vi "ActorDB-PerformUpdateAllInstruction.vi"(5 "SQL Statement":string, 6 "Cluster Out":T1(array[cluster]), 7 "Update All":bool, 8 "error in (no error)":errorcluster, 9 "Column Number":i32, 10 "Table":string, 11 "Database-API in":refnum<class "Database-API.lvclass">) -> (0 "Error Out":errorcluster[](array[cluster]), 3 "Database-API out":refnum<class "Database-API.lvclass">)   [LabVIEW 2013, in "Database-Actor.lvclass"]
uses:
  Database-Actor.lvclass
  Reuse Library/Database API/Database-API.lvclass
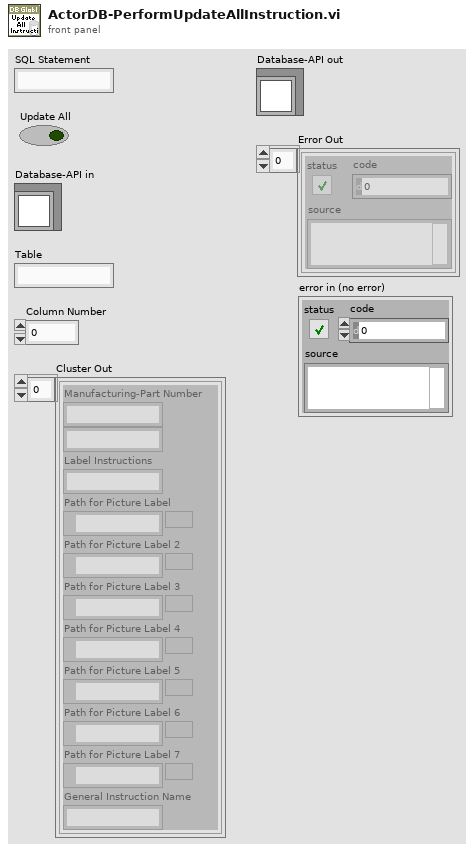
[diagram p1: front panel]
types:
  T1 = cluster{"Manufacturing-Part Number":string, string, "Label Instructions":string, "Path for Picture Label":path, "Path for Picture Label 2":path, "Path for Picture Label 3":path, "Path for Picture Label 4":path, "Path for Picture Label 5":path, "Path for Picture Label 6":path, "Path for Picture Label 7":path, "General Instruction Name":string}[]
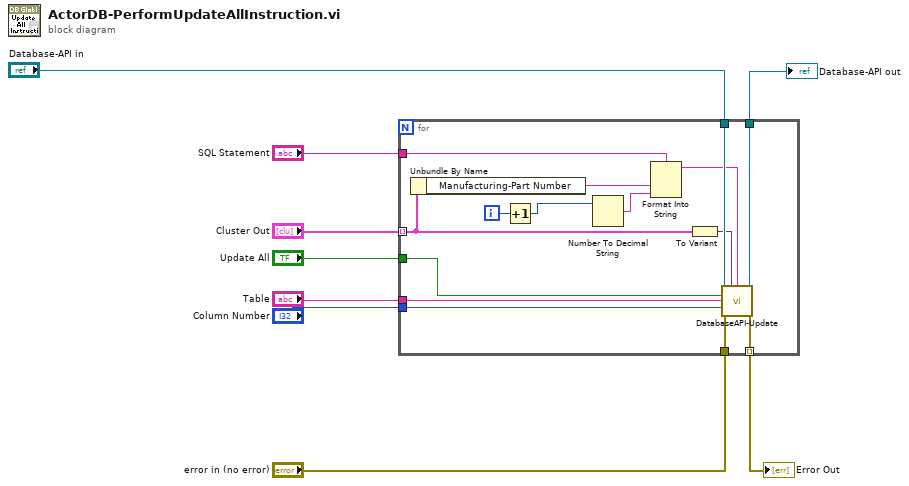
[diagram p0: block diagram]
diagram:
  n1 = for {
    tunnel: "Database-API in" -> [w24]
    tunnel: "Update All" -> [w23]
    tunnel: "SQL Statement" -> [w16]
    tunnel: [w22] -> w4
    tunnel: "Table" -> [w21]
    tunnel: [w20] -> w7 mode=indexing
    tunnel: "Column Number" -> [w19]
    tunnel: "error in (no error)" -> [w18]
    tunnel: "Cluster Out" -> [w15] mode=indexing
    i -> [w13]
    n2 = Unbundle By Name(w15) -> ("Manufacturing-Part Number"=w14:string)
    n3 = Increment(x=w13) -> (x+1=w12:i32)
    n4 = Number To Decimal String(number=w12) -> (decimal integer string=w11:string)  [unwired: 1 in]
    n5 = Format Into String(format string=w16, w14, w11) -> (resulting string=w10:string)  [unwired: 2 in, 1 out]
    n6 = To Variant(anything=w15) -> (Variant=w17:variant)
    n7 = call "DatabaseAPI-Update.vi"("Database-API in"=w24, "data"=w17, "Where Statement"=w10, "Update All"=w23, "Table"=w21, "Column Number"=w19, "error in (no error)"=w18) -> ("Database-API out"=w22:refnum<class "Database-API.lvclass">, "error out"=w20:errorcluster)  [unwired: 7 in]
  }
  "Error Out" <- w7
  "Database-API out" <- w4
